vi "Read GlobalConfiguration.vi"(11 "Template in":refnum<class "Template.lvclass">) -> (1 "ExecuteInterruptRoutine":bool, 2 "GlobalConfiguration":T1={"DeviceFamily"="", "WriteData"=FALSE, "BufferSize_samples"=-1, "SyncDevice"=FALSE, "ExecuteInterruptRoutine"=FALSE, "InterruptRoutineTimeout_ms"=-1}, 3 "InterruptRoutineTimeout":i32)   [LabVIEW 2020, in "Template.lvlib" / "Template.lvclass"]
doc: "Returns the global configuration from the configuration cluster"
uses:
  Template.lvclass
  typedefs/shared actor configuration.ctl
  Template.lvclass/Template.ctl
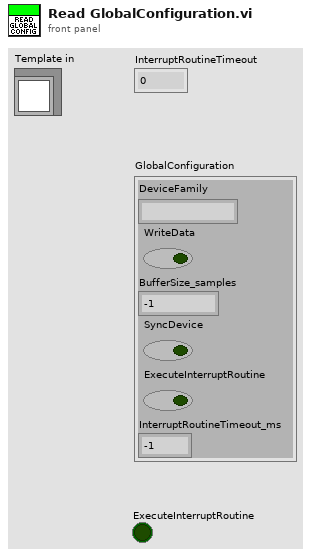
[diagram p1: front panel]
types:
  T1 = typedef "Template.lvlib/Template.lvclass/shared actor configuration.ctl" = cluster{"DeviceFamily":string, "WriteData":bool, "BufferSize_samples":i32, "SyncDevice":bool, "ExecuteInterruptRoutine":bool, "InterruptRoutineTimeout_ms":i32}
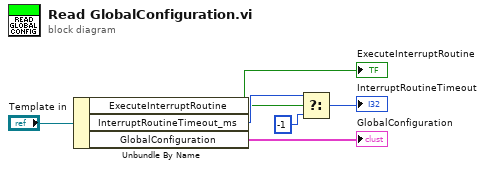
[diagram p0: block diagram]
diagram:
  n1 = Unbundle By Name("Template in") -> ("ExecuteInterruptRoutine"=w2:bool, "InterruptRoutineTimeout_ms"=w4:i32, "GlobalConfiguration"=→"GlobalConfiguration":T1)
  "ExecuteInterruptRoutine" <- w2
  n2 = Select(t=w4, s=w2, f=-1) -> (s? t:f=→"InterruptRoutineTimeout":i32)
